vi "QuantumDot Edit.vi"() -> ()   [LabVIEW 2019]
panel:
  out "Beta String":string
  in  "Write Time":dbl caption="Duration (ms)"
  in  "Write Voltage":dbl caption="Voltage"
  in  "Erase Time":dbl caption="Duration (ms)"
  in  "Erase Voltage":dbl caption="Voltage"
  in  "Write?":bool
  in  "Erase?":bool
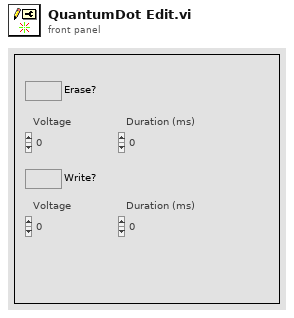
[diagram p1: front panel]
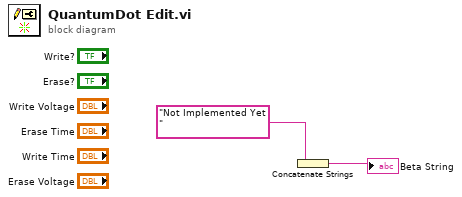
[diagram p0: block diagram]
diagram:
  n1 = Concatenate Strings("Not Implemented Yet ") -> (→"Beta String":string)
